vi "A_Vial RR Sub.vi"(7 "t":dbl, 8 "TotalTime":dbl, 9 "Vial Slope":dbl, 10 "Vial Temp":dbl, 11 "Param in":T1) -> (0 "Ave RR Down":dbl, 1 "Param out":T1, 3 "Ave RR Up":dbl)   [LabVIEW 2011]
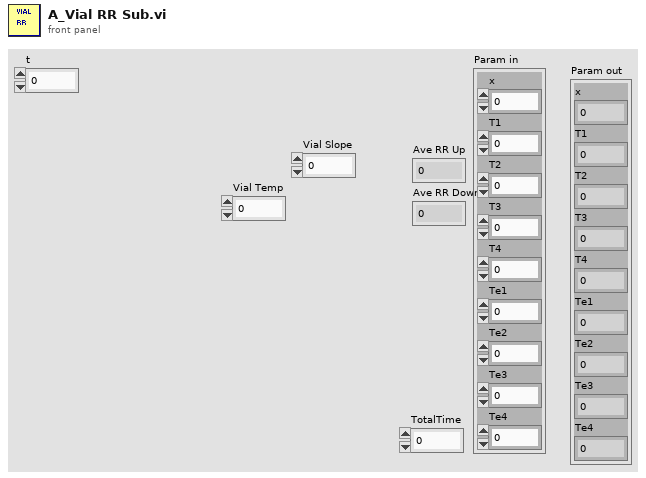
[diagram p1: front panel]
types:
  T1 = cluster{"x":dbl, "T1":dbl, "T2":dbl, "T3":dbl, "T4":dbl, "Te1":dbl, "Te2":dbl, "Te3":dbl, "Te4":dbl}
  T2 = cluster{"X":dbl, "T1":dbl, "T2":dbl, "T3":dbl, "T4":dbl, "Te1":dbl, "Te2":dbl, "Te3":dbl, "Te4":dbl}
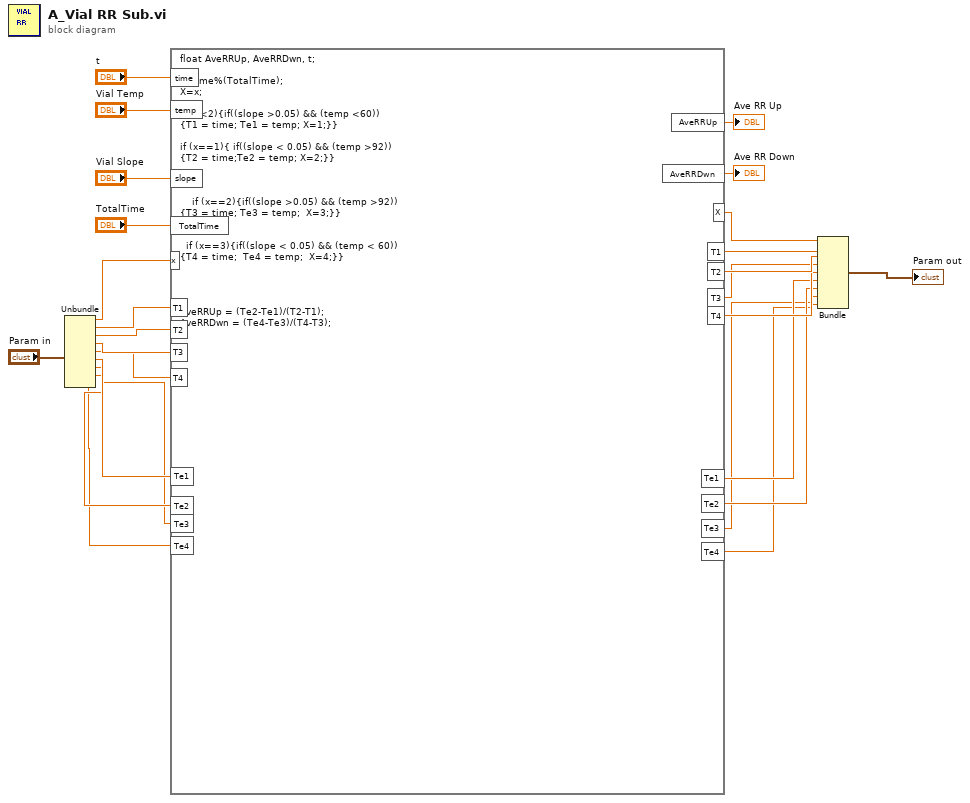
[diagram p0: block diagram]
diagram:
  n1 = Unbundle("Param in") -> ("x"=w10:dbl, "T1"=w9:dbl, "T2"=w8:dbl, "T3"=w7:dbl, "T4"=w6:dbl, "Te1"=w5:dbl, "Te2"=w4:dbl, "Te3"=w3:dbl, "Te4"=w2:dbl)
  n2 = formula code="float AveRRUp, AveRRDwn, t;\n\nt=time%(TotalTime);\nX=x;\n\n\tif (t<2){if((slope >0.05) && (temp <60))\n{T1 = time; Te1 = temp; X=1;}}\n\nif (x==1){ if((slope < 0.05) && (temp >92))\n{T2 = time;Te2 = temp; X=2;}}\n\t\t    \n\n\n\t\t\t if (x==2){if((slope >0.05) && (temp >92))\n{T3 = time; Te3 = temp; \tX=3;}}\n\n\n\t\tif (x==3){if((slope < 0.05) && (temp < 60))\n{T4 = time;  Te4 = temp; \tX=4;}}\n\n\n\t\t\t  \n\nAveRRUp = (Te2-Te1)/(T2-T1);\nAveRRDwn = (Te4-Te3)/(T4-T3);"("temp"="Vial Temp", "slope"="Vial Slope", "TotalTime"="TotalTime", "T1"=w9, "T2"=w8, "T3"=w7, "T4"=w6, "Te1"=w5, "Te2"=w4, "Te3"=w3, "Te4"=w2, "x"=w10, "time"="t") -> ("AveRRUp"=→"Ave RR Up":dbl, "AveRRDwn"=→"Ave RR Down":dbl, "X"=w21:dbl, "T1"=w20:dbl, "Te1"=w16:dbl, "Te2"=w15:dbl, "Te3"=w14:dbl, "Te4"=w13:dbl, "T2"=w19:dbl, "T3"=w18:dbl, "T4"=w17:dbl)
  n3 = Bundle("X"=w21, "T1"=w20, "T2"=w19, "T3"=w18, "T4"=w17, "Te1"=w16, "Te2"=w15, "Te3"=w14, "Te4"=w13) -> (→"Param out":T2)  [unwired: 1 in]
